vi "_PC_Tab set_layou.vi"(8 "error in (no error)":errorcluster, 11 "input cluster":T2) -> (0 "error out":errorcluster, 3 "tab ctrl refnums":T1)   [LabVIEW 2018]
uses:
  <vilib>/Utility/miscctls.llb/LVPositionTypeDef.ctl
  <vilib>/Utility/miscctls.llb/LVBoundsTypeDef.ctl
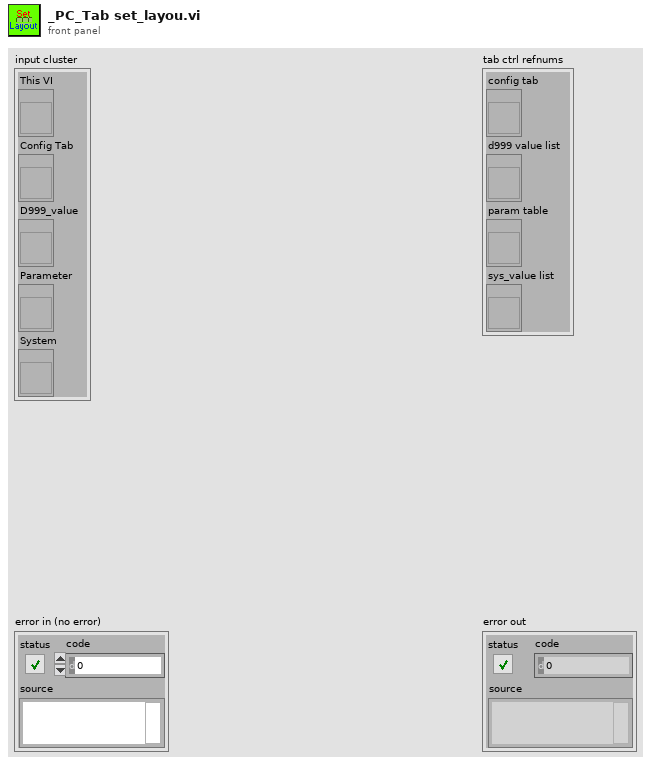
[diagram p1: front panel]
types:
  T1 = cluster{"config tab":refnum<vi>, "d999 value list":refnum<vi>, "param table":refnum<vi>, "sys_value list":refnum<vi>}
  T2 = cluster{"This VI":refnum<vi>, "Config Tab":refnum<vi>, "D999_value":refnum<vi>, "Parameter":refnum<vi>, "System":refnum<vi>}
  T3 = typedef "LVBoundsTypeDef.ctl" = cluster{"Width":u32, "Height":u32}
  T4 = typedef "LVPositionTypeDef.ctl" = cluster{"Left":i32, "Top":i32}
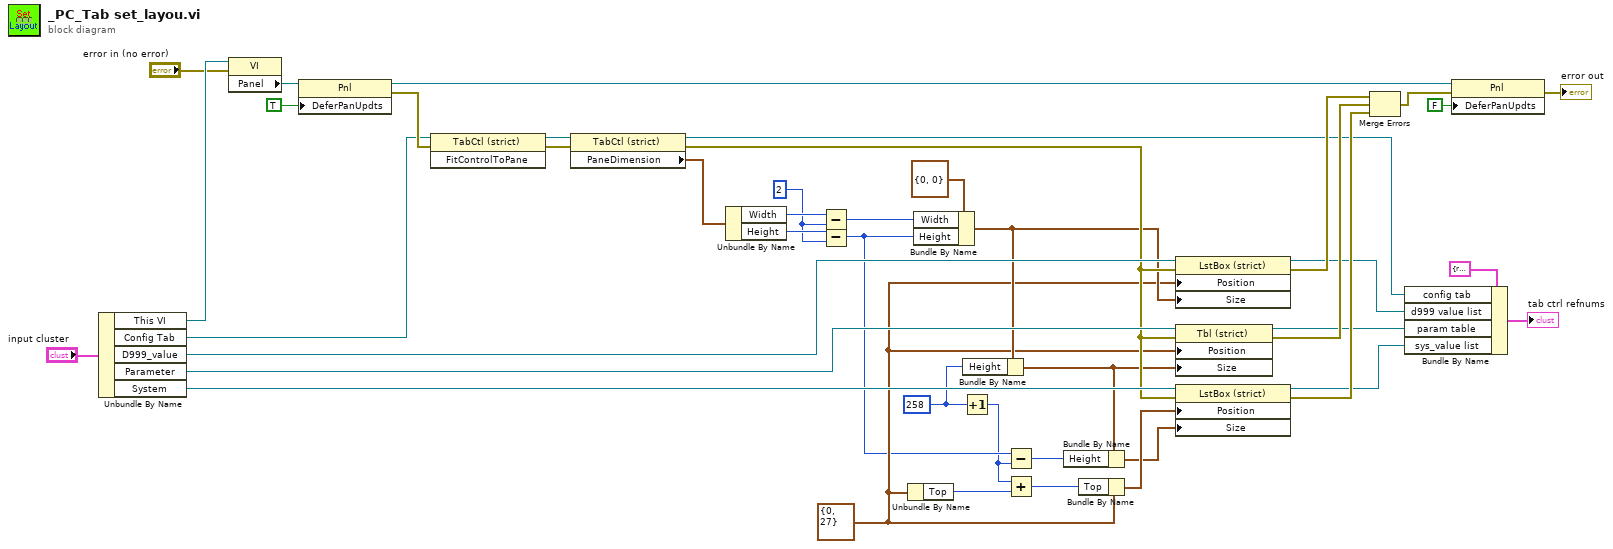
[diagram p0: block diagram]
diagram:
  w23 = u32 258 ("Height")
  w36 = u32 2 ("y")
  w25 = T4 {"Left"=0, "Top"=27} ("Position")
  n1 = Unbundle By Name("input cluster") -> ("This VI"=w33:refnum<vi>, "Config Tab"=w32:refnum<vi>, "D999_value"=w31:refnum<vi>, "Parameter"=w30:refnum<vi>, "System"=w29:refnum<vi>)
  n2 = property class="VI"(reference=w33, error in="error in (no error)") -> ("Panel"=w43:refnum<vi>)  [unwired: 2 out]
  n3 = property class="Pnl"(reference=w43, "DeferPanUpdts"=TRUE ("Defer Panel Updates")) -> (reference out=w15:refnum<vi>, error out=w41:errorcluster)  [unwired: 1 in]
  n4 = invoke class="TabCtl (strict)" method="FitControlToPane"(reference=w32, error in=w41) -> (reference out=w40:refnum<vi>, error out=w39:errorcluster)  [unwired: 1 in, 1 out]
  n5 = property class="TabCtl (strict)"(reference=w40, error in=w39) -> (reference out=w5:refnum<vi>, error out=w28:errorcluster, "PaneDimension"=w34:T3)
  n6 = Unbundle By Name(w34) -> ("Width"=w38:u32, "Height"=w37:u32)
  n7 = Subtract(x=w38, y=w36) -> (x-y=w35:u32)
  n8 = Subtract(x=w37, y=w36) -> (x-y=w20:u32)
  n9 = Unbundle By Name(w25) -> ("Top"=w22:i32)
  n10 = Bundle By Name(cluster=T3 {"Width"=0, "Height"=0} ("Size"), "Width"=w35, "Height"=w20) -> (w26:T3)
  n11 = Increment(x=w23) -> (x+1=w19:u32)
  n12 = Bundle By Name(cluster=w26, "Height"=w23) -> (w18:T3)
  n13 = Subtract(x=w20, y=w19) -> (x-y=w16:u32)
  n14 = Add(x=w19, y=w22) -> (x+y=w21:u32)
  n15 = Bundle By Name(cluster=w18, "Height"=w16) -> (w17:T3)
  n16 = Bundle By Name(cluster=w25, "Top"=w21) -> (w24:T4)
  n17 = property class="LstBox (strict)"(reference=w31, error in=w28, "Position"=w25, "Size"=w26) -> (reference out=w4:refnum<vi>, error out=w14:errorcluster)
  n18 = property class="Tbl (strict)"(reference=w30, error in=w28, "Position"=w25, "Size"=w18) -> (reference out=w3:refnum<vi>, error out=w13:errorcluster)
  n19 = property class="LstBox (strict)"(reference=w29, error in=w28, "Position"=w24, "Size"=w17) -> (reference out=w2:refnum<vi>, error out=w12:errorcluster)
  n20 = Merge Errors(w14, w13, w12) -> (w11:errorcluster)
  n21 = Bundle By Name(cluster=T1 {"config tab"=refnum, "d999 value list"=refnum, "param table"=refnum, "sys_value list"=refnum} ("tab ctrl refnums"), "config tab"=w5, "d999 value list"=w4, "param table"=w3, "sys_value list"=w2) -> (→"tab ctrl refnums":T1)
  n22 = property class="Pnl"(reference=w15, error in=w11, "DeferPanUpdts"=FALSE ("Defer Panel Updates")) -> (error out=→"error out":errorcluster)  [unwired: 1 out]
